vi "zad72.vi"() -> ()   [LabVIEW 2018]
uses:
  zad2states.ctl
panel:
  in  "?":bool
  in  "?":bool
  out "Pressed Numbers":string
  in  "?":bool
  in  "?":bool
  in  "?":bool
  in  "?":bool
  in  "?":bool
  in  "?":bool
  in  "?":bool
  in  "?":bool
  in  "?":bool
  in  "?":bool
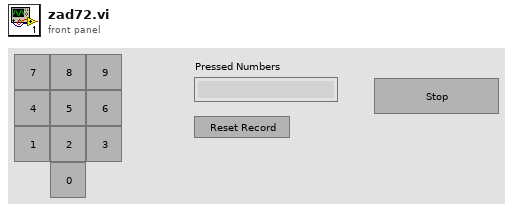
[diagram p1: front panel]
types:
  T1 = typedef "zad2states.ctl" = enum16{"Init", "ClearNumbers", "ReadingNumbers", "End"}
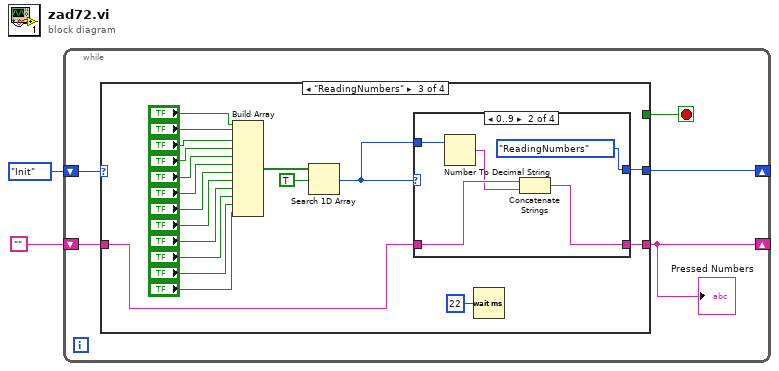
[diagram p0: block diagram]
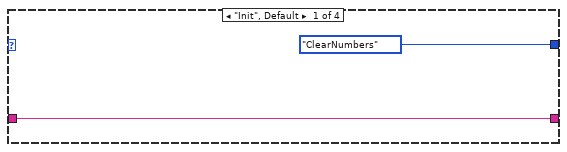
[diagram p2: hidden frame]
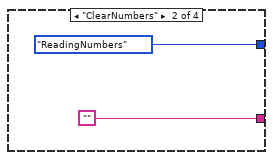
[diagram p3: hidden frame]
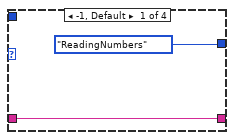
[diagram p4: hidden frame]
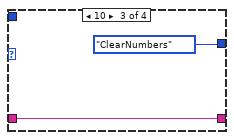
[diagram p5: hidden frame]
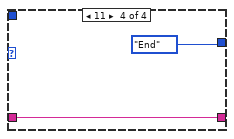
[diagram p6: hidden frame]
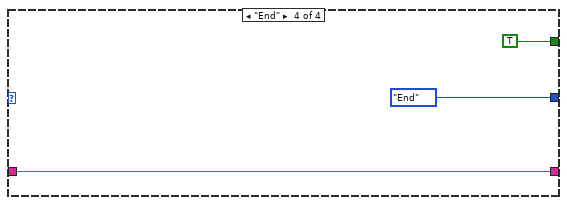
[diagram p7: hidden frame]
diagram:
  n1 = while {
    shift-right: [w5] -> _
    shift-left: zad2states."Init" -> [w7]
    shift-right: [w4] -> _
    shift-left: "" -> [w6]
    stop <- w3 stop-if-true
    n2 = case shown="\"ReadingNumbers\"" w7 {
      tunnel: w6 -> [w8 _ w17 w44]
      tunnel: [zad2states."ClearNumbers" zad2states."ReadingNumbers" w15 zad2states."End"] -> w5
      tunnel: [w8 "" w16 w44] -> w4
      tunnel: [_ _ _ TRUE] -> w3
      frame "Init", Default {
      }
      frame "ClearNumbers" {
      }
      frame "ReadingNumbers" {
        n3 = Build Array("?", "?", "?", "?", "?", "?", "?", "?", "?", "?", "?", "?") -> (w19:bool[])
        n4 = Search 1D Array(1D array=w19, element=TRUE) -> (index of element=w13:i32)  [unwired: 1 in]
        n5 = case shown="0..9" w13 {
          tunnel: w17 -> [w32 w36 w38 w40]
          tunnel: w13 -> [_ w37 _ _]
          tunnel: [w32 w34 w38 w40] -> w16
          tunnel: [zad2states."ReadingNumbers" zad2states."ReadingNumbers" zad2states."ClearNumbers" zad2states."End"] -> w15
          frame -1, Default {
          }
          frame 0..9 {
            n6 = Number To Decimal String(number=w37) -> (decimal integer string=w35:string)  [unwired: 1 in]
            n7 = Concatenate Strings(w36, w35) -> (w34:string)
          }
          frame 10 {
          }
          frame 11 {
          }
        }
        n8 = Wait (ms)(milliseconds to wait=u32 22) -> ()  [unwired: 1 out]
      }
      frame "End" {
      }
    }
    "Pressed Numbers" <- w4
  }
